vi "GetText.vi"(8 "error in":errorcluster, 11 "Module Editor Node in":refnum<class "module editor node.lvclass">) -> (0 "error out":errorcluster, 1 "additional text":string, 2 "text":string, 3 "Module Editor Node out":refnum<class "module editor node.lvclass">, 4 "glyph":string)   [LabVIEW 2013, in "PL Framework Configuration Tool.lvlib" / "module editor node.lvclass"]
uses:
  module editor node.lvclass
  TBM Configuration Node/TBM Configuration Node.lvclass
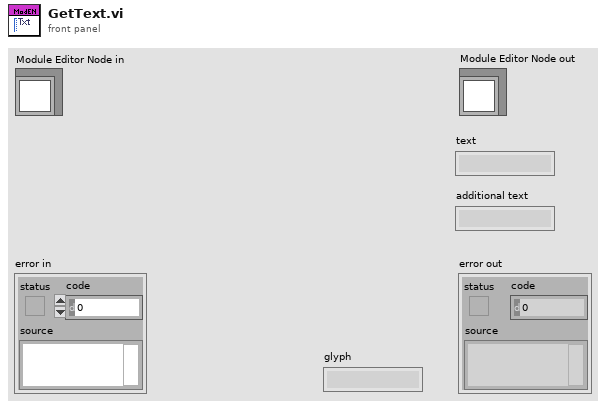
[diagram p1: front panel]
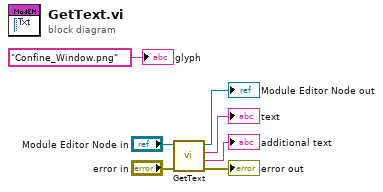
[diagram p0: block diagram]
diagram:
  n1 = call-parent "GetText.vi"("error in"="error in", "node in"="Module Editor Node in") -> ("error out"=→"error out":errorcluster, "additional text"=→"additional text":string, "text"=→"text":string, "node out"=→"Module Editor Node out":refnum<class "module editor node.lvclass">)  [unwired: 5 in, 1 out]
  "glyph" <- "Confine_Window.png" ("glyph")
